vi "Settings.vi"(4 "Component Tray ID":i32, 6 "Baseplate Tray ID":i32, 7 "Glue step":enum16{"Kapton", "Sensor", "PCB"}(ring), 8 "error in (no error)":errorcluster, 9 "Gantry Region":i32=1, 10 "Tray ID":i32=1, 11 "Syringe Space in":refnum<class "Syringe Space.lvclass">) -> (0 "error out":errorcluster, 3 "Syringe Space out":refnum<class "Syringe Space.lvclass">)   [LabVIEW 2016, in "Syringe Space.lvclass"]
uses:
  Syringe Space.lvclass
  C:/Users/HEP Gantry/Documents/GitHub/UCSB-Gantry/V5/Classes/Workspace/Fixture.lvclass
  C:/Users/HEP Gantry/Documents/GitHub/UCSB-Gantry/V5/Classes/Workspace/Carrier Tray/Assembly Tray.lvclass
  Fixture.lvclass/Fixture.ctl
  Assembly Tray.lvclass/Assembly Tray.ctl
  Write Fixture ID.vi
  Write Syringe.vi
  Write Gantry Region.vi
panel:
  # "Syringe Space"
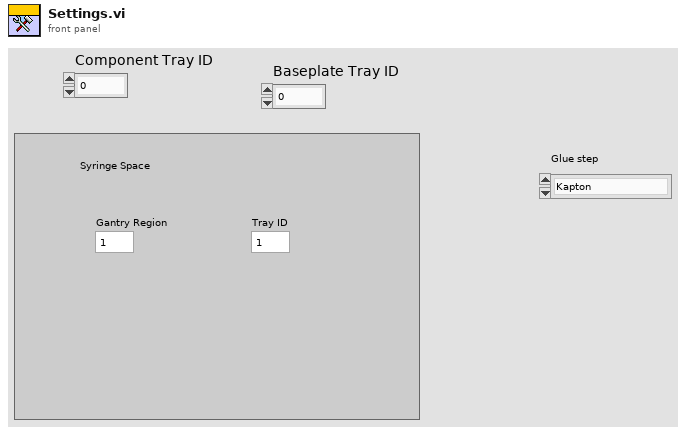
[diagram p1: front panel]
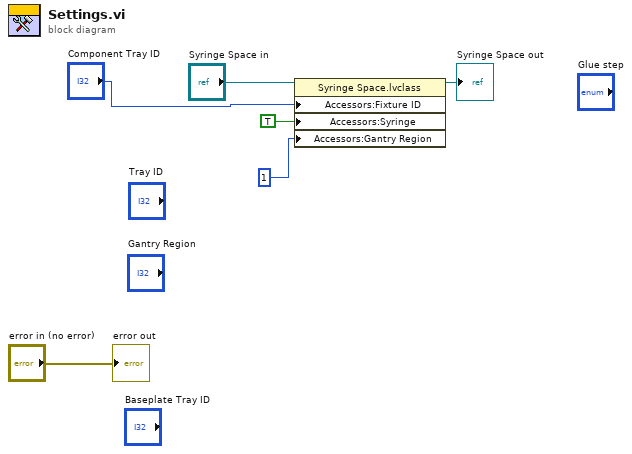
[diagram p0: block diagram]
diagram:
  n1 = property class="Syringe Space.lvclass"(reference="Syringe Space in", "Accessors:Fixture ID"="Component Tray ID", "Accessors:Syringe"=TRUE ("Syringe"), "Accessors:Gantry Region"=1) -> (reference out=→"Syringe Space out":refnum<class "Syringe Space.lvclass">)  [unwired: 1 in, 1 out]
  "error out" <- "error in (no error)"
